vi "CheckDisplacementTimeout.vi"(11 "DisplacementData in":T1) -> (3 "DisplacementData out":T1)   [LabVIEW 2016]
uses:
  DisplacementData.ctl
  DisplacementStates.ctl
  DisplacementSample.ctl
  DisplacementErrorSample.ctl
  DisplacementErrorCodes.ctl
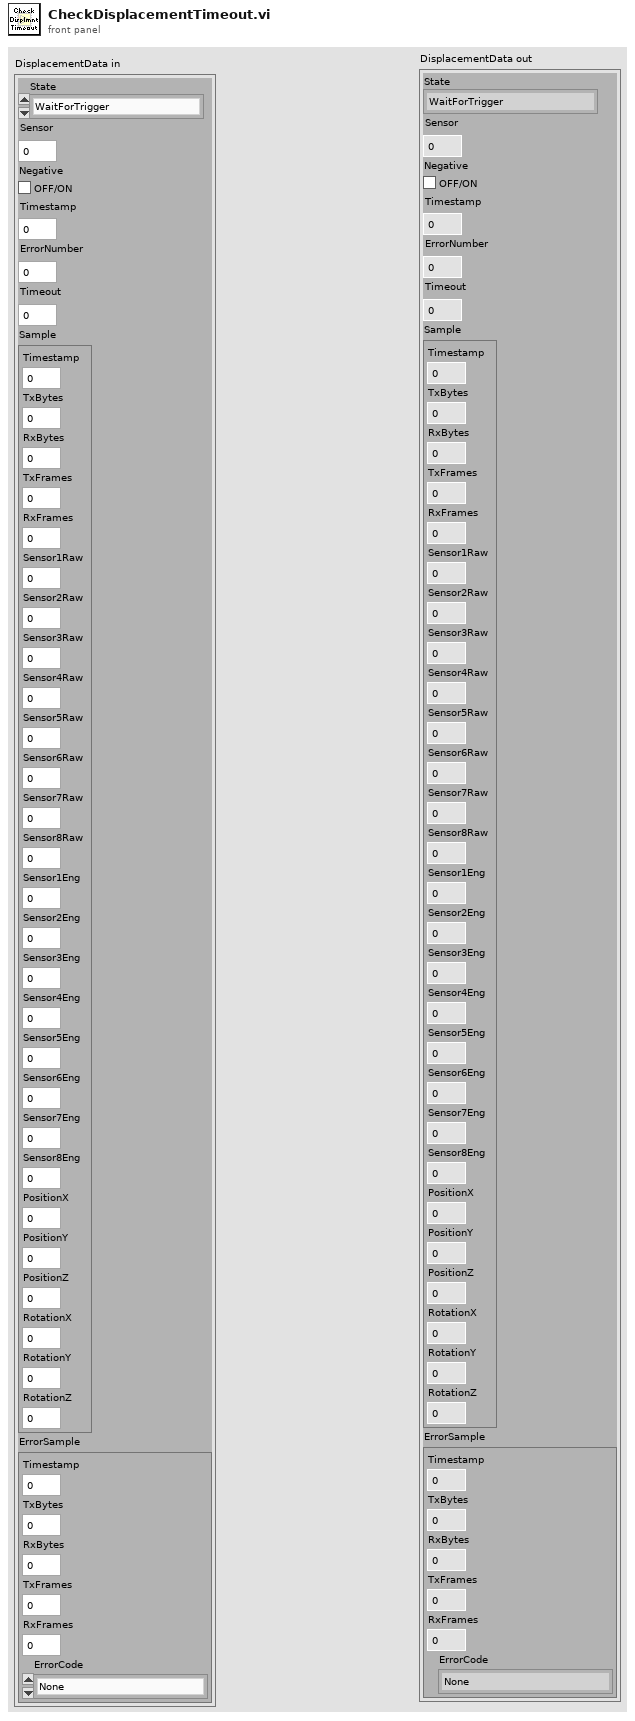
[diagram p1: front panel]
types:
  T1 = typedef "DisplacementData.ctl" = cluster{"State":T2, "Sensor":u8, "Negative":bool, "Timestamp":u64, "ErrorNumber":u8, "Timeout":i32, "Sample":T3, "ErrorSample":T4}
  T2 = typedef "DisplacementStates.ctl" = enum16{"WaitForTrigger", "ClearRxFIFO", "WaitForClearComplete", "WriteM", "Write0", "WriteCR", "WriteNL", "ReadFirstCharacter", "ReadDataResponse", "ReadDeliminator", "ReadSign", "ReadHundreds", "ReadTens", "ReadOnes", "ReadDecimal", "ReadTenths", "ReadHundredths", "ReadThousandths", "ReadTenThousandths", "PrepareSample", "MoveSample", "ReadErrorR", "ReadErrorDeliminator1", "ReadErrorM", "ReadError0", "ReadErrorDeliminator2", "ReadErrorNumberTens", "ReadErrorNumberOnes", "ReadErrorCR", "ParseErrorNumber", "ResponseUnknownError", "ResponseInvalidError", "ResponseTimeoutError", "SensorIndicatesInvalidCommandError", "SensorIndicatesCommunicationTimeoutError", "SensorIndicatesDataLengthError", "SensorIndicatesNumberOfParametersError", "SensorIndicatesParameterError", "SensorIndicatesCommunicationError", "SensorIndicatesIDNumberError", "SensorIndicatesExpansionLineError", "SensorIndicatesWriteControlError", "PrepareErrorCode", "MoveErrorCode"}
  T3 = typedef "DisplacementSample.ctl" = cluster{"Timestamp":u64, "TxBytes":u64, "RxBytes":u64, "TxFrames":u64, "RxFrames":u64, "Sensor1Raw":i32, "Sensor2Raw":i32, "Sensor3Raw":i32, "Sensor4Raw":i32, "Sensor5Raw":i32, "Sensor6Raw":i32, "Sensor7Raw":i32, "Sensor8Raw":i32, "Sensor1Eng":sgl, "Sensor2Eng":sgl, "Sensor3Eng":sgl, "Sensor4Eng":sgl, "Sensor5Eng":sgl, "Sensor6Eng":sgl, "Sensor7Eng":sgl, "Sensor8Eng":sgl, "PositionX":sgl, "PositionY":sgl, "PositionZ":sgl, "RotationX":sgl, "RotationY":sgl, "RotationZ":sgl}
  T4 = typedef "DisplacementErrorSample.ctl" = cluster{"Timestamp":u64, "TxBytes":u64, "RxBytes":u64, "TxFrames":u64, "RxFrames":u64, "ErrorCode":T5}
  T5 = typedef "DisplacementErrorCodes.ctl" = enum16{"None", "ResponseUnknownError", "ResponseInvalidError", "ResponseTimeoutError", "SensorIndicatesInvalidCommandError", "SensorIndicatesCommunicationTimeoutError", "SensorIndicatesDataLengthError", "SensorIndicatesNumberOfParametersError", "SensorIndicatesParameterError", "SensorIndicatesCommunicationError", "SensorIndicatesIDNumberError", "SensorIndicatesExpansionLineError", "SensorIndicatesWriteControlError"}
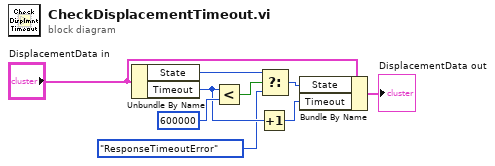
[diagram p0: block diagram]
diagram:
  n1 = Unbundle By Name("DisplacementData in") -> ("State"=w1:T2, "Timeout"=w7:i32)
  n2 = Less?(x=w7, y=600000) -> (x < y?=w8:bool)
  n3 = Increment(x=w7) -> (x+1=w2:i32)
  n4 = Select(t=w1, s=w8, f=DisplacementStates."ResponseTimeoutError") -> (s? t:f=w3:T2)
  n5 = Bundle By Name(cluster="DisplacementData in", "State"=w3, "Timeout"=w2) -> (→"DisplacementData out":T1)
